vi "GetText.vi"(8 "error in":errorcluster, 11 "node in":refnum<class "NISE_CEF_Node.lvclass">) -> (0 "error out":errorcluster, 1 "additional text":string, 2 "text":string, 3 "node out":refnum<class "NISE_CEF_Node.lvclass">, 4 "glyph":string)   [LabVIEW 2013, in "NISE_CEF_Node.lvclass"]
doc: "Returns the text representation of the node used for the tree control."
uses:
  NISE_CEF_Node.lvclass
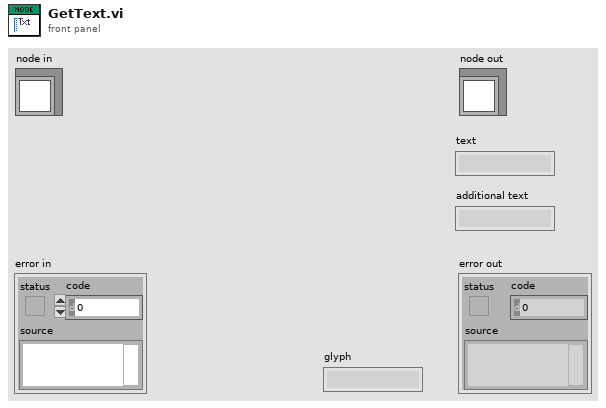
[diagram p1: front panel]
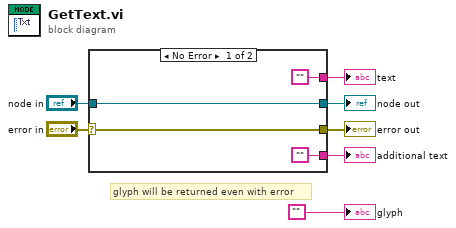
[diagram p0: block diagram]
diagram:
  # "glyph will be returned even with error"
  n1 = case shown="No Error" "error in" {
    selector: "error in" -> [w10 w13]
    tunnel: [w10 w13] -> w6
    tunnel: [w11 w12] -> w4
    tunnel: "node in" -> [w11 w12]
    tunnel: ["" _] -> w3
    tunnel: ["" _] -> w2
    frame No Error {
    }
    frame Error {
    }
  }
  "error out" <- w6
  "node out" <- w4
  "text" <- w3
  "additional text" <- w2
  "glyph" <- ""
